vi "User_Panel Appear.vi"(8 "error in (no error)":errorcluster caption="错误输入（无错误）") -> (0 "error out":errorcluster caption="错误输出")   [LabVIEW 2020]
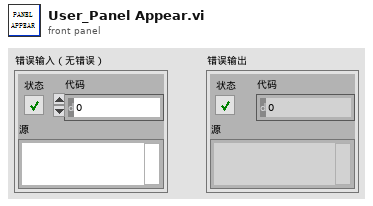
[diagram p1: front panel]
types:
  T1 = enum32{"Invalid", "Standard", "Closed", "Hidden", "Minimized", "Maximized"}
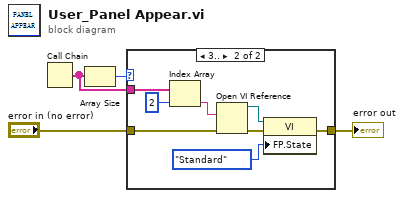
[diagram p0: block diagram]
diagram:
  n1 = Call Chain() -> (call chain=w2:string[])
  n2 = Array Size(array=w2) -> (size(s)=w1:i32)
  n3 = case shown="3.." w1 {
    tunnel: "error in (no error)" -> [w5 w8]
    tunnel: [w5 w7] -> w3
    tunnel: w2 -> [_ w6]
    frame 0, Default {
    }
    frame 3.. {
      n4 = Index Array(array=w6, index=2 ("索引")) -> (element=w11:string)
      n5 = Open VI Reference(vi path=w11, error in (no error)=w8) -> (vi reference=w12:refnum<vi>, error out=w13:errorcluster)  [unwired: 4 in]
      n6 = property class="VI"(reference=w12, error in=w13, "FP.State"=T1."Standard" ("前面板窗口:状态")) -> (error out=w7:errorcluster)  [unwired: 1 out]
    }
  }
  "error out" <- w3
